vi "CommonVIs_CreateBD-StringConstantDocumentation.vi"(7 "App":refnum<vi>, 8 "error in (no error)":errorcluster, 9 "Remove extra prefixed spaces on every row but keep indentation":bool, 10 "Documentation":string, 11 "VI Ref/Vi Path":variant) -> (0 "error out":errorcluster)   [LabVIEW 2012]
uses:
  <vilib>/Utility/traverseref.llb/TRef TravTarget.ctl
  <vilib>/Utility/miscctls.llb/LVPointTypeDef.ctl
  <vilib>/Utility/traverseref.llb/VI Scripting - Traverse.lvlib
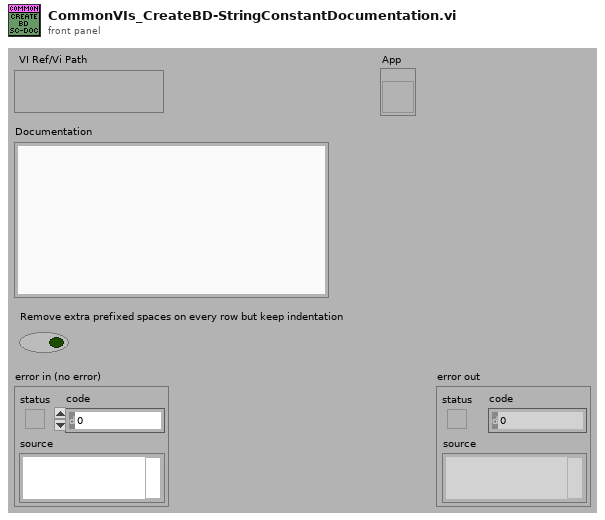
[diagram p1: front panel]
types:
  T1 = typedef "TRef TravTarget.ctl" = enum16{"FP", "BD", "Other"}
  T2 = typedef "LVPointTypeDef.ctl" = cluster{"Horizontal":i16, "Vertical":i16}
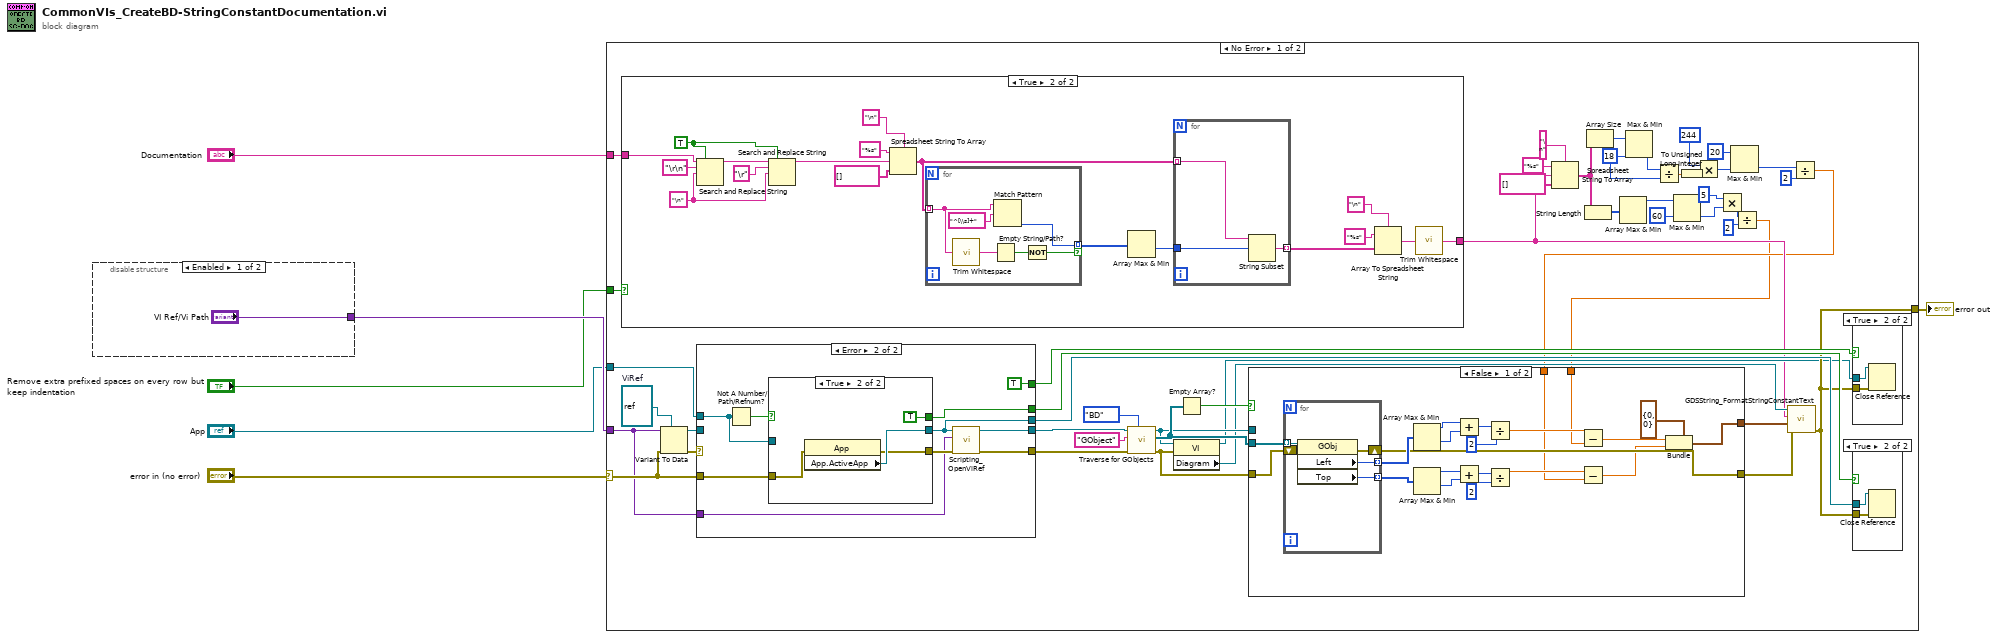
[diagram p0: block diagram]
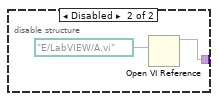
[diagram p2: hidden frame]
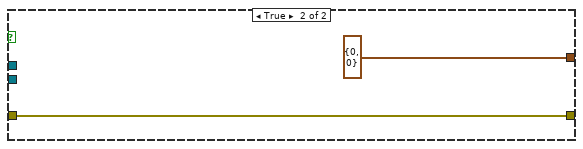
[diagram p4: hidden frame]
diagram:
  n1 = disable-structure shown="Enabled" {
    disable-tunnel: ["VI Ref/Vi Path" w9] -> w4
    frame Enabled {
    }
    frame Disabled {
      n2 = Open VI Reference(vi path=path "E:/LabVIEW/A.vi") -> (vi reference=w9:refnum<vi>)  [unwired: 5 in, 1 out]
    }
  }
  n3 = case shown="No Error" "error in (no error)" {
    selector: "error in (no error)" -> [w53 w136]
    tunnel: [w49 w136] -> w5
    tunnel: w4 -> [w35 _]
    tunnel: "App" -> [w54 _]
    tunnel: "Documentation" -> [w37 _]
    tunnel: "Remove extra prefixed spaces on every row but keep indentation" -> [w36 _]
    frame No Error {
      w28 = 18 ("y")
      w56 = refnum<vi> refnum  # ViRef
      n4 = case shown="True" w36 {
        tunnel: w37 -> [w58 w60]
        tunnel: [w58 w59] -> w29
        frame False {
        }
        frame True {
          w63 = "\n" ("search string")
          w64 = TRUE ("replace all? (F)")
          n5 = Search and Replace String(replace all?=w64, input string=w60, search string="\r\n", replace string=w63) -> (result string=w66:string)  [unwired: 4 in, 3 out]
          n6 = Search and Replace String(replace all?=w64, input string=w66, search string="\r", replace string=w63) -> (result string=w62:string)  [unwired: 4 in, 3 out]
          n7 = Spreadsheet String To Array(delimiter (Tab)="\n", format string="%s" ("spreadsheet string"), spreadsheet string=w62, array type (2D Dbl)=string[] []) -> (array=w72:string[])
          n8 = for {
            tunnel: w72 -> [w83] mode=indexing
            tunnel: [w84] -> w73 mode=indexing if=w80
            n9 = call <vilib>:"Trim Whitespace.vi"("string"=w83) -> ("trimmed string"=w82:string)  [unwired: 1 in]
            n10 = Empty String/Path?(string/path=w82) -> (empty?=w81:bool)
            n11 = Match Pattern(string=w83, regular expression="^[\\s]+") -> (offset past match=w84:i32)  [unwired: 1 in, 3 out]
            n12 = Not(x=w81) -> (.not. x?=w80:bool)
          }
          n13 = Array Max & Min(array=w73) -> (min value=w71:i32)  [unwired: 3 out]
          n14 = for {
            tunnel: w72 -> [w79] mode=indexing
            tunnel: w71 -> [w78]
            tunnel: [w77] -> w70 mode=indexing
            n15 = String Subset(string=w79, offset (0)=w78) -> (substring=w77:string)  [unwired: 1 in]
          }
          n16 = Array To Spreadsheet String(delimiter (Tab)="\n", array=w70, 3:"%s" ("spreadsheet string")) -> (spreadsheet string=w61:string)
          n17 = call <vilib>:"Trim Whitespace.vi"("string"=w61) -> ("trimmed string"=w59:string)  [unwired: 1 in]
        }
      }
      n18 = Variant To Data(error in=w53, type=w56, Variant=w35) -> (data=w55:refnum<vi>, error out=w57:errorcluster)
      n19 = case shown="Error" w57 {
        selector: w57 -> [w118 _]
        tunnel: [w119 w129] -> w45
        tunnel: w55 -> [w119 _]
        tunnel: w53 -> [_ w127]
        tunnel: [w118 w126] -> w48
        tunnel: w54 -> [_ w124]
        tunnel: [_ TRUE] -> w52
        tunnel: [_ w122] -> w51
        tunnel: [_ w121] -> w50
        tunnel: w35 -> [_ w120]
        frame No Error {
        }
        frame Error {
          n20 = Not A Number/Path/Refnum?(number/path/refnum=w124) -> (NaN/Path/Refnum?=w125:bool)
          n21 = case shown="True" w125 {
            tunnel: [w131 w135] -> w121
            tunnel: [w130 w134] -> w128
            tunnel: w127 -> [w130 w133]
            tunnel: w124 -> [w131 _]
            tunnel: [_ TRUE] -> w122
            frame False {
            }
            frame True {
              n22 = property class="App"(error in=w133) -> (error out=w134:errorcluster, "App.ActiveApp"=w135:refnum<vi>)  [unwired: 1 in, 1 out]
            }
          }
          n23 = call <resource>:"Scripting_OpenViRef.vi"("error in"=w128, "ViPath/ViName"=w120, "AppRef"=w121) -> ("error out"=w126:errorcluster, "vi reference"=w129:refnum<vi>)  [unwired: 7 in]
        }
      }
      n24 = call <vilib>:"Traverse for GObjects.vi"("Traverse Target"=TRef_TravTarget."BD", "error in (no error)"=w48, "Class Name"="GObject", "VI Refnum"=w45) -> ("error out"=w38:errorcluster, "References"=w44:refnum<vi>[], "dup VI Refnum"=w42:refnum<vi>)  [unwired: 4 in, 1 out]
      n25 = property class="VI"(reference=w42, error in=w38) -> (reference out=w41:refnum<vi>, "Diagram"=w40:refnum<vi>)  [unwired: 1 out]
      n26 = Empty Array?(array=w44) -> (empty?=w43:bool)
      n27 = Spreadsheet String To Array(delimiter (Tab)="\n", format string="%s", spreadsheet string=w29, array type (2D Dbl)=string[] []) -> (array=w18:string[])
      n28 = String Length(string=w18) -> (length=w21:i32[])
      n29 = Array Size(array=w18) -> (size(s)=w31:i32)
      n30 = Array Max & Min(array=w21) -> (max value=w20:i32)  [unwired: 3 out]
      n31 = Max & Min(x=w31, y=w28) -> (min(x,y)=w27:i32)  [unwired: 1 out]
      n32 = Divide(x=w27, y=w28) -> (x/y=w26:dbl)
      n33 = Max & Min(x=w20, y=60) -> (min(x,y)=w11:i32)  [unwired: 1 out]
      n34 = To Unsigned Long Integer(number=w26) -> (unsigned 32bit integer=w22:u32)
      n35 = Multiply(x=u32 244 ("Height"), y=w22) -> (x*y=w24:u32)
      n36 = Multiply(x=5, y=w11) -> (x*y=w10:i32)
      n37 = Max & Min(x=u32 20, y=w24) -> (min(x,y)=w16:u32)  [unwired: 1 out]
      n38 = Divide(x=w10, y=u32 2 ("x")) -> (x/y=w13:dbl)
      n39 = Divide(x=w16, y=u32 2 ("x")) -> (x/y=w14:dbl)
      n40 = case shown="False" w43 {
        tunnel: w44 -> [w105 _]
        tunnel: w42 -> [_ _]
        tunnel: w38 -> [w101 w112]
        tunnel: [w102 T2 {"Horizontal"=0, "Vertical"=0} ("location")] -> w39
        tunnel: [w100 w112] -> w34
        tunnel: w14 -> [w87 _]
        tunnel: w13 -> [w86 _]
        frame False {
          n41 = for {
            tunnel: w105 -> [w111] mode=indexing
            tunnel: [w110] -> w106 mode=indexing
            tunnel: [w109] -> w104 mode=indexing
            shift-right: [w107] -> w100
            shift-left: w101 -> [w108]
            n42 = property class="GObj"(reference=w111, error in=w108) -> (error out=w107:errorcluster, "Left"=w110:i32, "Top"=w109:i32)  [unwired: 1 out]
          }
          n43 = Array Max & Min(array=w106) -> (max value=w99:i32, min value=w98:i32)  [unwired: 2 out]
          n44 = Array Max & Min(array=w104) -> (max value=w94:i32, min value=w93:i32)  [unwired: 2 out]
          n45 = Add(x=w99, y=w98) -> (x+y=w97:i32)
          n46 = Add(x=w94, y=w93) -> (x+y=w95:i32)
          n47 = Divide(x=w97, y=2) -> (x/y=w91:dbl)
          n48 = Divide(x=w95, y=2) -> (x/y=w88:dbl)
          n49 = Subtract(x=w91, y=w86) -> (x-y=w90:dbl)
          n50 = Subtract(x=w88, y=w87) -> (x-y=w89:dbl)
          n51 = Bundle(cluster=T2 {"Horizontal"=0, "Vertical"=0} ("location"), "Horizontal"=w90, "Vertical"=w89) -> (w102:T2)
        }
        frame True {
        }
      }
      n52 = call <resource>:"GDSString_FormatStringConstantText.vi"("error in (no error)"=w34, "location"=w39, "StringConstantText"=w29, "StringConstantOwner"=w40) -> ("error out"=w49:errorcluster)  [unwired: 7 in]
      n53 = case shown="True" w52 {
        tunnel: w41 -> [_ w117]
        tunnel: w49 -> [_ w116]
        frame False {
        }
        frame True {
          n54 = Close Reference(reference=w117, error in (no error)=w116) -> ()  [unwired: 1 out]
        }
      }
      n55 = case shown="True" w51 {
        tunnel: w50 -> [_ w115]
        tunnel: w49 -> [_ w114]
        frame False {
        }
        frame True {
          n56 = Close Reference(reference=w115, error in (no error)=w114) -> ()  [unwired: 1 out]
        }
      }
    }
    frame Error {
    }
  }
  "error out" <- w5
